vi "Verify new image.vi"(8 "error in (no error)":errorcluster, 11 "CCDCamera in":refnum<class "CCDCamera.lvclass">) -> (0 "error out":errorcluster, 2 "New Images ?":bool, 3 "CCDCamera out":refnum<class "CCDCamera.lvclass">)   [LabVIEW 2018, in "CCDCamera.lvclass"]
doc: "Verifies if there is any new image"
uses:
  CCDCamera.lvclass
  C:/Users/observer/Desktop/SPARC4_ACS/SPARC4_ACS/Simulated_CCD_Camera/Simulated_CCD_Camera.lvclass
  Simulated_CCD_Camera/Simulated_CCD_Camera.lvclass
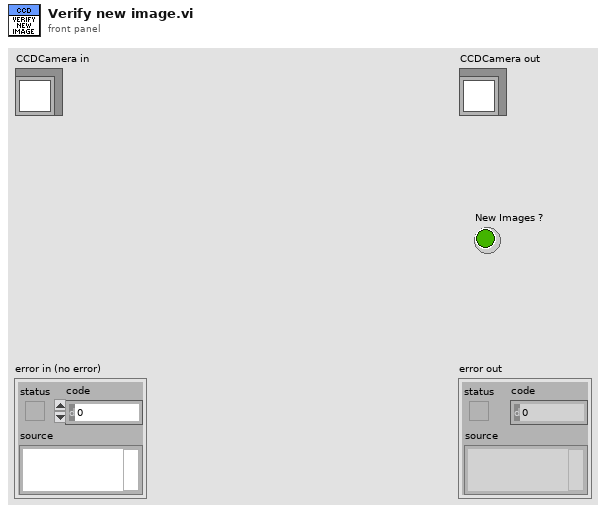
[diagram p1: front panel]
types:
  T1 = cluster{"CYCLES_DONE":u16, "LAST_IMAGE_NAME":string, "DISK_SPACE":u16, "FRAMES_DONE":u16, "CCD_STATUS":string, "CURRENT_TEMPERATURE":i16, "TEMPERATURE_STATUS":string, "FRAME_EXPOSURE_TIME":sgl, "ERROR":bool, "SERIAL_NUMBER":u16, "ACQUIRING":bool, "IMAGE_INDEX":u32, "SEQS_DONE":u16}
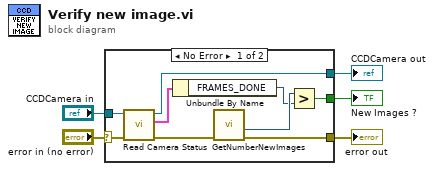
[diagram p0: block diagram]
diagram:
  n1 = case shown="No Error" "error in (no error)" {
    selector: "error in (no error)" -> [w8 w16]
    tunnel: [w13 w16] -> w4
    tunnel: [w10 w15] -> w2
    tunnel: "CCDCamera in" -> [w11 w15]
    tunnel: [w12 _] -> w1
    frame No Error {
      n2 = call "Read Camera Status.vi"("error in (no error)"=w8, "CCDCamera in"=w11) -> ("error out"=w9:errorcluster, "Camera Status"=w7:T1, "CCDCamera out"=w10:refnum<class "CCDCamera.lvclass">)  [unwired: 7 in]
      n3 = Unbundle By Name(w7) -> ("FRAMES_DONE"=w6:u16)
      n4 = call <userlib>:"GetNumberNewImages.vi"("error in (no error)"=w9) -> ("error out"=w13:errorcluster, "last"=w14:i32)  [unwired: 3 in, 2 out]
      n5 = Greater?(x=w14, y=w6) -> (0:w12:bool)
    }
    frame Error {
    }
  }
  "error out" <- w4
  "CCDCamera out" <- w2
  "New Images ?" <- w1
